vi "FRCts20_Backend_Dyn_GetSglTeam.vi"(6 "Message Attributes":T4, 8 "error in (no error)":errorcluster, 10 "Data":string, 11 "Engine_Refnums":T1) -> (0 "error out":errorcluster)   [LabVIEW 2014, in "FRCts20_Backend_DynamicLoad.lvlib"]
uses:
  FRCts20_Backend_DynamicLoad.lvlib
  Dependencies/Keyed Array/KeyedArray.ctl
  Dependencies/Keyed Array/Tools_KeyedArray.lvlib
  Dependencies/AMC/_SubVIs/TypeDefs/Message.ctl
  Dependencies/AMC/AMC.lvlib
  Dependencies/AMC/_SubVIs/TypeDefs/Message Queue.ctl
  FRCts20_Backend_EngineRefnums.ctl
  FRCts20_Backend_Engine.lvlib
  <vilib>/addons/database/Connection.llb/Conn ObjectReference.ctl
  <vilib>/addons/database/NI_Database_API.lvlib
  INI_Accessor/FRCts20_Backend_INI Controller.lvclass
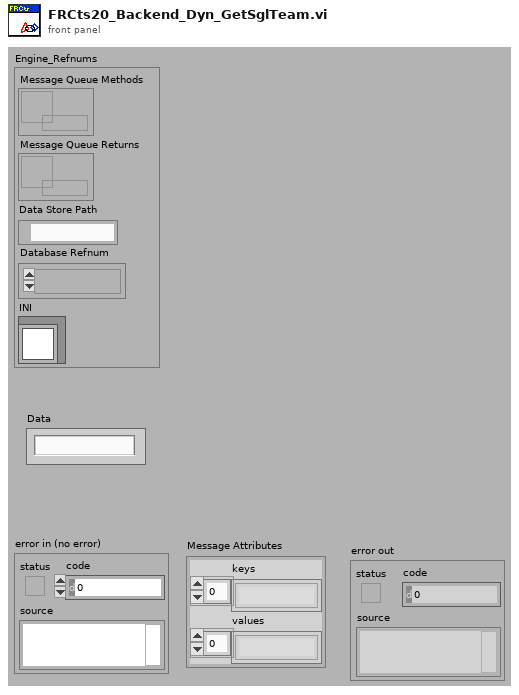
[diagram p1: front panel]
types:
  T1 = typedef "FRCts20_Backend_Engine.lvlib/FRCts20_Backend_EngineRefnums.ctl" = cluster{"Message Queue Methods":T2, "Message Queue Returns":T2, "Data Store Path":path, "Database Refnum":T3, "INI":refnum<class "FRCts20_Backend_INI Controller.lvclass">}
  T2 = typedef "AMC.lvlib/Message Queue.ctl" = refnum<queue>
  T3 = typedef "NI_Database_API.lvlib/Conn ObjectReference.ctl" = refnum<k1>
  T4 = typedef "Tools_KeyedArray.lvlib/KeyedArray.ctl" = cluster{"keys":string[], "values":string[]}
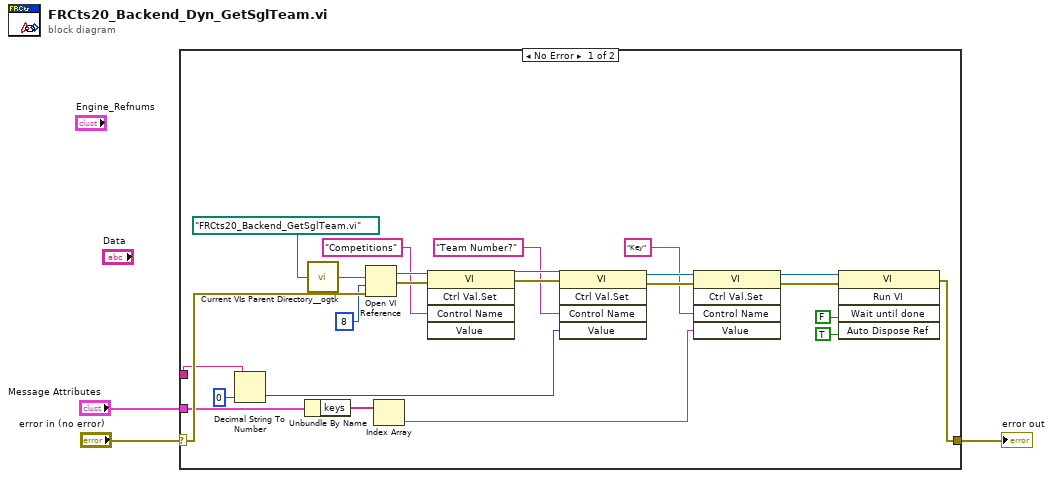
[diagram p0: block diagram]
diagram:
  n1 = case shown="No Error" "error in (no error)" {
    selector: "error in (no error)" -> [w26 w29]
    tunnel: [w17 w29] -> w3
    tunnel: [w10 _] -> w2
    tunnel: "Message Attributes" -> [w7 _]
    frame No Error {
      n2 = Decimal String To Number(string=w10, default (0L)=u16 0) -> (number=w8:u16)  [unwired: 1 in, 1 out]
      n3 = Unbundle By Name(w7) -> ("keys"=w6:string[])
      n4 = call "Current VIs Parent Directory__ogtk.vi"("Relative path (.)"=path "FRCts20_Backend_GetSglTeam.vi") -> ("Parent Directory (+ Relative)"=w27:path)  [unwired: 4 in]
      n5 = Open VI Reference(vi path=w27, options=8, error in (no error)=w26) -> (vi reference=w25:refnum<vi>, error out=w24:errorcluster)  [unwired: 3 in]
      n6 = Index Array(array=w6) -> (element=w5:string)  [unwired: 1 in]
      n7 = invoke class="VI" method="Ctrl Val.Set"(reference=w25, error in=w24, "Control Name"="Competitions") -> (reference out=w22:refnum<vi>, error out=w21:errorcluster)  [unwired: 2 in, 3 out]
      n8 = invoke class="VI" method="Ctrl Val.Set"(reference=w22, error in=w21, "Control Name"="Team Number?", "Value"=w8) -> (reference out=w16:refnum<vi>, error out=w15:errorcluster)  [unwired: 1 in, 3 out]
      n9 = invoke class="VI" method="Ctrl Val.Set"(reference=w16, error in=w15, "Control Name"="Key", "Value"=w5) -> (reference out=w13:refnum<vi>, error out=w12:errorcluster)  [unwired: 1 in, 3 out]
      n10 = invoke class="VI" method="Run VI"(reference=w13, error in=w12, "Wait until done"=FALSE ("Wait Until Done"), "Auto Dispose Ref"=TRUE ("Auto Dispose Reference")) -> (error out=w17:errorcluster)  [unwired: 1 in, 4 out]
    }
    frame Error {
    }
  }
  "error out" <- w3
